vi "MuxCardSwitch.vi"(6 "Single Needle":bool, 7 "Probe Card Channels":i32=32, 8 "error in (no error)":errorcluster, 9 "disabled channels":u32[](array[numeric]), 10 "Switch to channel":i32, 11 "LXIPXISwitching in":refnum<class "LXIPXISwitching.lvclass">) -> (0 "error out":errorcluster, 2 "last channel no.":i32, 3 "LXIPXISwitching out":refnum<class "LXIPXISwitching.lvclass">)   [LabVIEW 2019, in "LXIPXISwitching.lvclass"]
uses:
  LXIPXISwitching.lvclass
  Switching.lvclass
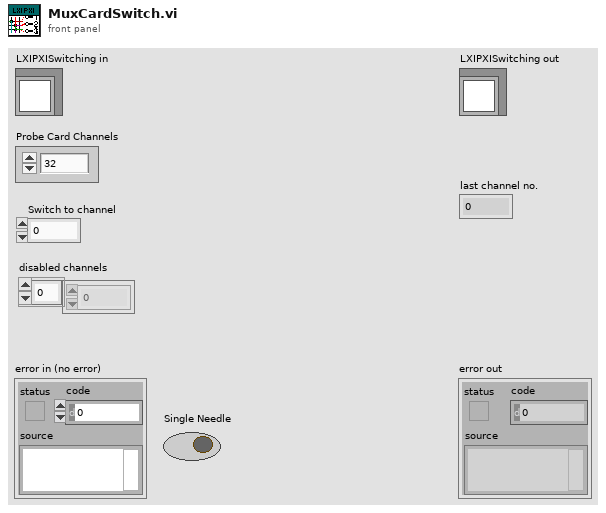
[diagram p1: front panel]
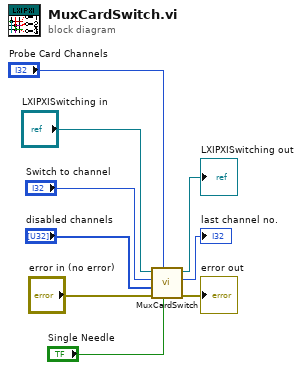
[diagram p0: block diagram]
diagram:
  n1 = call-parent "MuxCardSwitch.vi"("Single Needle"="Single Needle", "Probe Card Channels"="Probe Card Channels", "error in (no error)"="error in (no error)", "disabled channels"="disabled channels", "Switch to channel"="Switch to channel", "Switching in"="LXIPXISwitching in") -> ("error out"=→"error out":errorcluster, "last channel no."=→"last channel no.":i32, "Switching out"=→"LXIPXISwitching out":refnum<class "LXIPXISwitching.lvclass">)  [unwired: 3 in]
